vi "GetDouble.vi"(8 "error in (no error)":errorcluster, 11 "MsgPackDeserializer in":refnum<class "MsgPackDeserializer.lvclass">) -> (0 "error out":errorcluster, 2 "Number":dbl format="%.2f", 3 "MsgPackDeserializer out":refnum<class "MsgPackDeserializer.lvclass">)   [LabVIEW 2015, in "MsgPackDeserializer.lvclass"]
uses:
  MsgPackDeserializer.lvclass
  MsgPackDeserializer.lvclass/MsgPackDeserializer.ctl
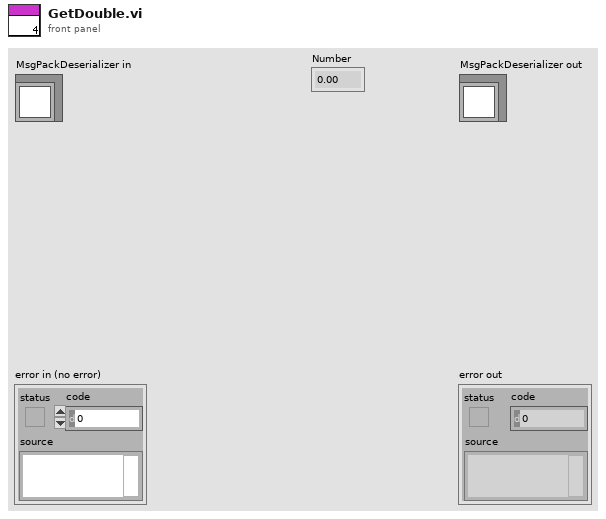
[diagram p1: front panel]
types:
  T1 = enum16{"big-endian, network order", "native, host order", "little-endian"}
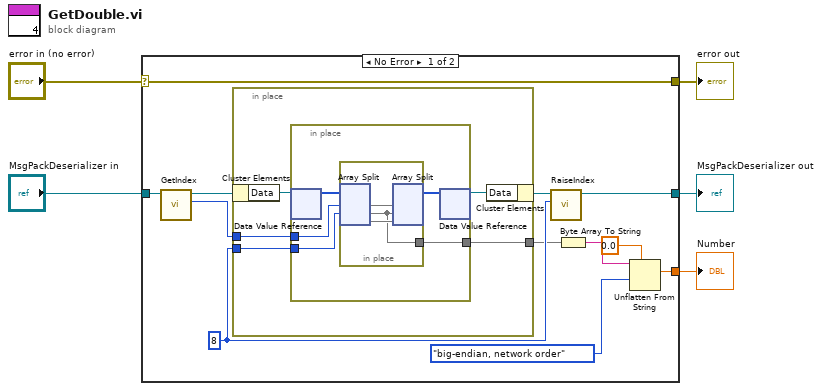
[diagram p0: block diagram]
diagram:
  n1 = case shown="No Error" "error in (no error)" {
    selector: "error in (no error)" -> [w17 w32]
    tunnel: [w17 w32] -> w4
    tunnel: [w13 w31] -> w2
    tunnel: "MsgPackDeserializer in" -> [w16 w31]
    tunnel: [w6 _] -> w1
    frame No Error {
      w11 = i64 8 ("x")
      n2 = call "GetIndex.vi"("MsgPackDeserializer in"=w16) -> ("Index"=w14:i64, "MsgPackDeserializer out"=w15:refnum<class "MsgPackDeserializer.lvclass">)  [unwired: 8 in, 1 out]
      n3 = in-place {
        in-place-border: w14 -> [w21]
        in-place-border: w11 -> [w19]
        in-place-border: [w18] -> w10
        n4 = in-place-cluster #1(w15) -> ("Data"=w20:refnum<data-value>)
        n5 = in-place {
          in-place-border: w21 -> [w26]
          in-place-border: w19 -> [w25]
          in-place-border: [w23] -> w18
          n6 = in-place-dvr #2(w20) -> (w27:u8[])  [unwired: 1 out]
          n7 = in-place {
            in-place-border: [w28] -> w23
            n8 = in-place-split #3(w27, w26, w25) -> (w30:u8[], w28:u8[], w29:u8[])
            n9 = in-place-split #3(w30, w28, w29) -> (w24:u8[])  [unwired: 2 out]
          }
          n10 = in-place-dvr #2(w24) -> (w22:refnum<data-value>)  [unwired: 1 out]
        }
        n11 = in-place-cluster #1("Data"=w22) -> (w12:refnum<class "MsgPackDeserializer.lvclass">)
      }
      n12 = call "RaiseIndex.vi"("x"=w11, "MsgPackDeserializer in"=w12) -> ("MsgPackDeserializer out"=w13:refnum<class "MsgPackDeserializer.lvclass">)  [unwired: 8 in, 1 out]
      n13 = Byte Array To String(unsigned byte array=w10) -> (string=w9:string)
      n14 = Unflatten From String(type=0.0 ("x"), binary string=w9, byte order (0:big-endian, network order)=T1."big-endian, network order") -> (value=w6:dbl)  [unwired: 2 in, 2 out]
    }
    frame Error {
    }
  }
  "error out" <- w4
  "MsgPackDeserializer out" <- w2
  "Number" <- w1
